vi "New Layout (instant).vi"(6 "wait for reply (T)":bool=TRUE, 8 "error in (no error)":errorcluster, 10 "Cage parameters":variant) -> (0 "error out":errorcluster, 1 "timed out?":bool, 2 "Reply Payload":T1)   [LabVIEW 2018, in "Cage Diagram.lvlib"]
doc: "The same as New Layout, but with instant reply instead of broadcast.\n_____\nCreated using Delacor QMH Event Scripter 4.2.1.88."
uses:
  Cage Diagram.lvlib
  New Layout (instant) (Reply Payload)--cluster.ctl
  <vilib>/vision/Image Controls.llb/IMAQ Image.ctl
  SubVi's/Controls/CTL_Pixel_to_Zone_array.ctl
  Typedefs/CTL_Cage_drawing_params.ctl
  SubVi's/Controls/CTL_Draw_Area_Size.ctl
  Typedefs/CTL_Cage_External_dimensions.ctl
  Typedefs/CTL_Image_Scaling_info.ctl
  SubVi's/Controls/CTL_Segments_Colors_(pie).ctl
  New Layout (instant) Argument--cluster.ctl
  Common_Resources.lvlib
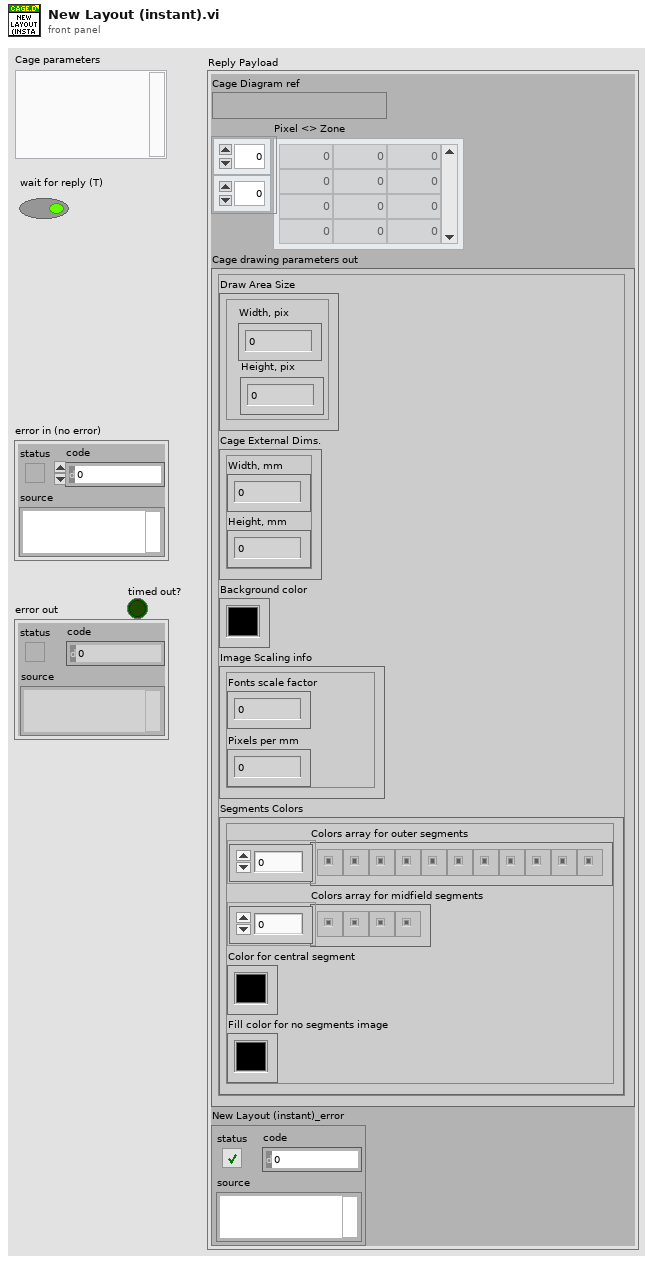
[diagram p1: front panel]
types:
  T1 = typedef "Cage Diagram.lvlib/New Layout (instant) (Reply Payload)--cluster.ctl" = cluster{"Cage Diagram ref":T2, "Pixel <> Zone":T3, "Cage drawing parameters out":T4, "New Layout (instant)_error":errorcluster}
  T2 = typedef "IMAQ Image.ctl" = refnum<image>
  T3 = typedef "Common_Resources.lvlib/CTL_Pixel_to_Zone_array.ctl" = i8[][]
  T4 = typedef "Cage Diagram.lvlib/CTL_Cage_drawing_params.ctl" = cluster{"Draw Area Size":T5, "Cage External Dims.":T6, "Background color":u32, "Image Scaling info":T7, "Segments Colors":T8}
  T5 = typedef "Common_Resources.lvlib/CTL_Draw_Area_Size.ctl" = cluster{"Width, pix":i32, "Height, pix":i32}
  T6 = typedef "Cage Diagram.lvlib/CTL_Cage_External_dimensions.ctl" = cluster{"Width, mm":dbl, "Height, mm":dbl}
  T7 = typedef "Cage Diagram.lvlib/CTL_Image_Scaling_info.ctl" = cluster{"Fonts scale factor":dbl, "Pixels per mm":dbl}
  T8 = typedef "Common_Resources.lvlib/CTL_Segments_Colors_(pie).ctl" = cluster{"Colors array for outer segments":u32[], "Colors array for midfield segments":u32[], "Color for central segment":u32, "Fill color for no segments image":u32}
  T9 = typedef "Cage Diagram.lvlib/New Layout (instant) Argument--cluster.ctl" = cluster{"Cage parameters":variant, "Wait Notifier":refnum<notifier>, "wait for reply":bool}
  T10 = typedef "Cage Diagram.lvlib/Request Events--cluster.ctl" = cluster{"Stop Module":refnum<user-event>, "Show Panel":refnum<user-event>, "Hide Panel":refnum<user-event>, "Get Module Execution Status":refnum<user-event>, "Show Diagram":refnum<user-event>, "New Layout":refnum<user-event>, "New Layout (instant)":refnum<user-event>}
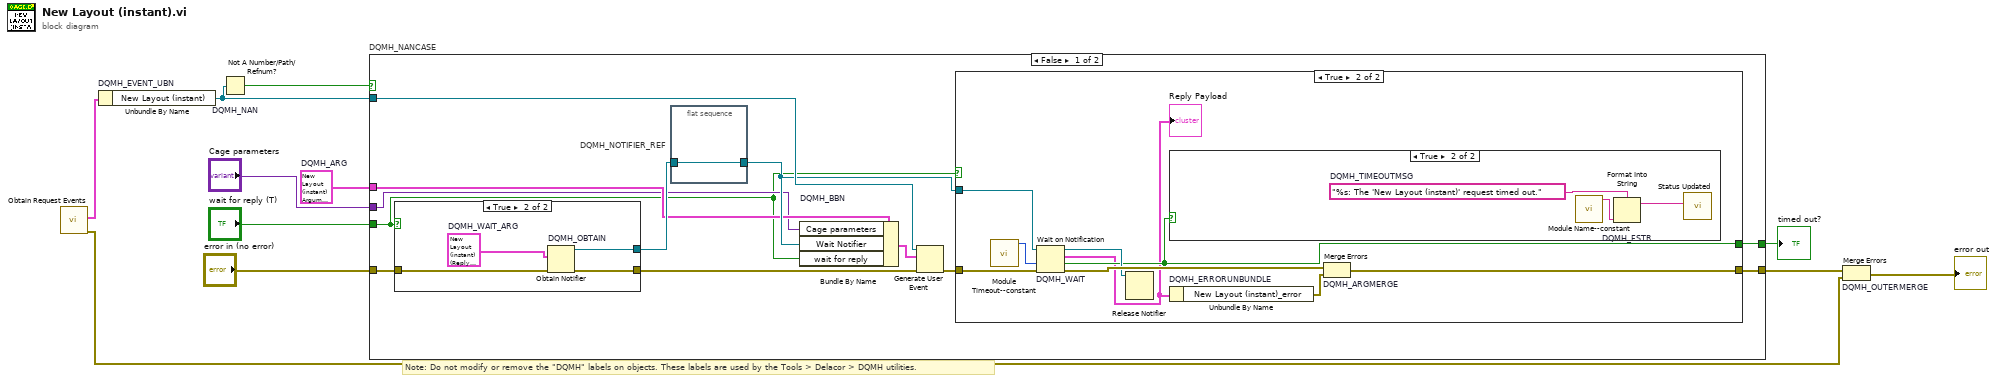
[diagram p0: block diagram]
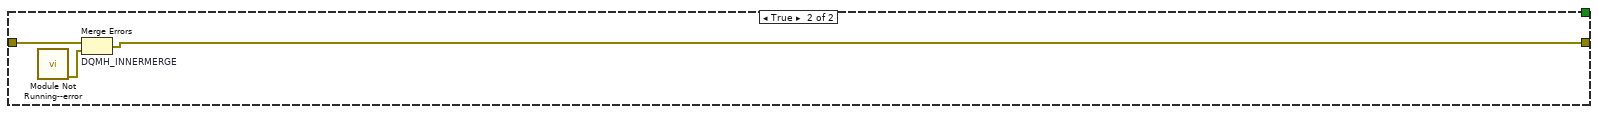
[diagram p5: hidden frame]
diagram:
  w5 = T9 {"Cage parameters"=variant, "Wait Notifier"=refnum, "wait for reply"=FALSE}  # DQMH_ARG
  # "Note: Do not modify or remove the \"DQMH\" labels on objects. These labels are used by the Tools > Delacor > DQMH utilities."
  n1 = call "Obtain Request Events.vi"() -> ("error out"=w2:errorcluster, "Cage Diagram Request Events"=w1:T10)  [unwired: 10 in]
  n2 = Unbundle By Name "DQMH_EVENT_UBN"(w1) -> ("New Layout (instant)"=w9:refnum<user-event>)
  n3 = Not A Number/Path/Refnum? "DQMH_NAN"(number/path/refnum=w9) -> (NaN/Path/Refnum?=w8:bool)
  n4 = case "DQMH_NANCASE" shown="False" w8 {
    tunnel: "error in (no error)" -> [w23 w45]
    tunnel: w9 -> [w21 _]
    tunnel: [w18 w44] -> w6
    tunnel: [w19 _] -> w7
    tunnel: w5 -> [w14 _]
    tunnel: "Cage parameters" -> [w13 _]
    tunnel: "wait for reply (T)" -> [w12 _]
    frame False {
      n5 = case shown="True" w12 {
        tunnel: w23 -> [w38 w42]
        tunnel: [w38 w41] -> w20
        tunnel: [_ w39] -> w16
        frame False {
        }
        frame True {
          w40 = T1 {"Cage Diagram ref"=refnum, "Pixel <> Zone"=[], "Cage drawing parameters out"={"Draw Area Size"={"Width, pix"=0, "Height, pix"=0}, "Cage External Dims."={"Width, mm"=0.0, "Height, mm"=0.0}, "Background color"=0, "Image Scaling info"={"Fonts scale factor"=0.0, "Pixels per mm"=0.0}, "Segments Colors"={"Colors array for outer segments"=[], "Colors array for midfield segments"=[], "Color for central segment"=0, "Fill color for no segments image"=0}}, "New Layout (instant)_error"={"status"=FALSE, "code"=0, "source"=""}}  # DQMH_WAIT_ARG
          n6 = Obtain Notifier "DQMH_OBTAIN"(notification data type=w40, error in (no error)=w42) -> (notifier out=w39:refnum<notifier>, error out=w41:errorcluster)  [unwired: 2 in, 1 out]
        }
      }
      n7 = flat-sequence "DQMH_NOTIFIER_REF" {
        tunnel: w16 -> [w24]
        tunnel: [w24] -> w15
        frame #0 {
        }
      }
      n8 = Bundle By Name "DQMH_BBN"(cluster=w14, "Cage parameters"=w13, "Wait Notifier"=w15, "wait for reply"=w12) -> (w17:T9)
      n9 = Generate User Event(user event=w21, event data cluster=w17, error in=w20) -> (error out=w22:errorcluster)  [unwired: 1 in, 1 out]
      n10 = case shown="True" w12 {
        tunnel: w22 -> [w25 w34]
        tunnel: w15 -> [_ w32]
        tunnel: [_ w30] -> w19
        tunnel: [w25 w29] -> w18
        frame False {
        }
        frame True {
          n11 = call "Module Timeout--constant.vi"() -> ("Module Timeout"=w26:i32)  [unwired: 11 in]
          n12 = Wait on Notification "DQMH_WAIT"(notifier=w32, timeout in ms (-1)=w26, error in (no error)=w34) -> (notifier out=w31:refnum<notifier>, notification=w27:T1, timed out?=w30:bool, error out=w33:errorcluster)  [unwired: 1 in]
          "Reply Payload" <- w27
          n13 = Release Notifier(notifier=w31) -> ()  [unwired: 2 in, 3 out]
          n14 = case shown="True" w30 {
            frame False {
            }
            frame True {
              w37 = "%s: The 'New Layout (instant)' request timed out."  # DQMH_TIMEOUTMSG
              n15 = call "Module Name--constant.vi"() -> ("Module Name"=w36:string)  [unwired: 11 in]
              n16 = Format Into String "DQMH_FSTR"(format string=w37, w36) -> (resulting string=w35:string)  [unwired: 2 in, 1 out]
              n17 = call "Status Updated.vi"("Status"=w35) -> ()  [unwired: 10 in, 1 out]
            }
          }
          n18 = Unbundle By Name "DQMH_ERRORUNBUNDLE"(w27) -> ("New Layout (instant)_error"=w28:errorcluster)
          n19 = Merge Errors "DQMH_ARGMERGE"(w33, w28) -> (w29:errorcluster)
        }
      }
    }
    frame True {
      n20 = call "Module Not Running--error.vi"() -> ("error out"=w43:errorcluster)  [unwired: 11 in]
      n21 = Merge Errors "DQMH_INNERMERGE"(w45, w43) -> (w44:errorcluster)
    }
  }
  "timed out?" <- w7
  n22 = Merge Errors "DQMH_OUTERMERGE"(w6, w2) -> (→"error out":errorcluster)
